vi "Master_ActuatorStates.vi"(8 "error in (no error)":errorcluster) -> (0 "error out":errorcluster, 2 "CurrentActuations":T1={"Pod Power"=FALSE, "Dump Valve"=TRUE, "Brakes"=FALSE, "Clamp"=FALSE, "Pump"=FALSE, "Ignition"=FALSE, "DO6"=FALSE, "DO7"=FALSE, "HighSide"=FALSE, "Precharge"=FALSE, "LowSide"=FALSE, "DO3"=FALSE, "DO4"=FALSE, "DO5"=FALSE, "DO62"=FALSE, "DO72"=FALSE})   [LabVIEW 2018]
doc: "Reads state of actuators and formats it for data stream."
uses:
  Control/TypeDef_DigitalOuts.ctl
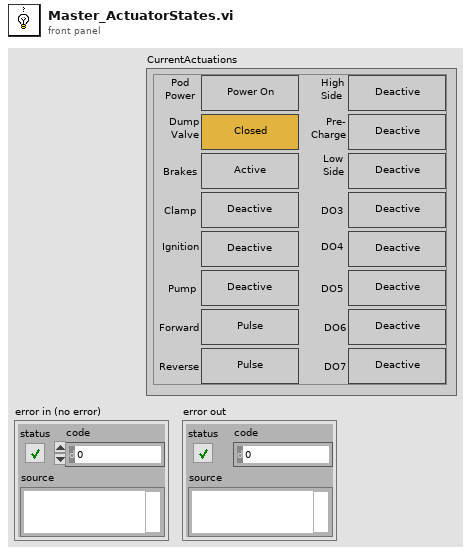
[diagram p1: front panel]
types:
  T1 = typedef "TypeDef_DigitalOuts.ctl" = cluster{"Pod Power":bool, "Dump Valve":bool, "Brakes":bool, "Clamp":bool, "Pump":bool, "Ignition":bool, "DO6":bool, "DO7":bool, "HighSide":bool, "Precharge":bool, "LowSide":bool, "DO3":bool, "DO4":bool, "DO5":bool, "DO62":bool, "DO72":bool}
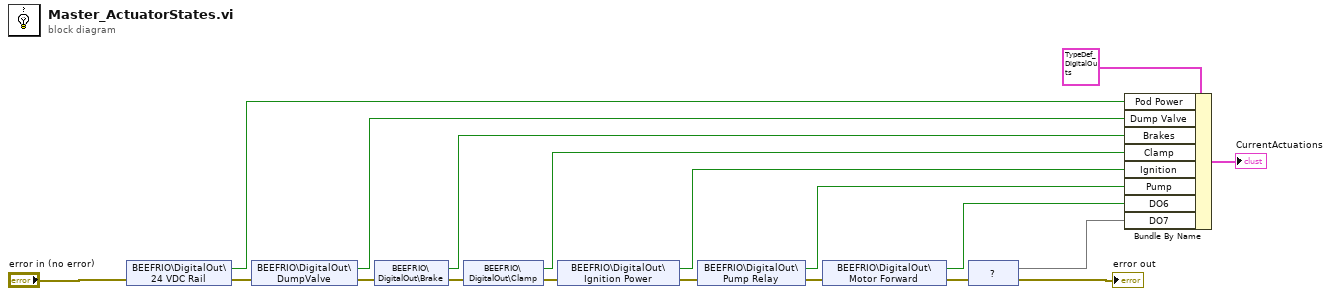
[diagram p0: block diagram]
diagram:
  n1 = shared-variable "BEEFRIO\\DigitalOut\\24 VDC Rail"(error in="error in (no error)") -> (w8:bool, error out=w19:errorcluster)
  n2 = shared-variable "BEEFRIO\\DigitalOut\\DumpValve"(error in=w19) -> (w7:bool, error out=w18:errorcluster)
  n3 = shared-variable "BEEFRIO\\DigitalOut\\Brake"(error in=w18) -> (w6:bool, error out=w17:errorcluster)
  n4 = shared-variable "BEEFRIO\\DigitalOut\\Clamp"(error in=w17) -> (w5:bool, error out=w13:errorcluster)
  n5 = shared-variable "BEEFRIO\\DigitalOut\\Ignition Power"(error in=w13) -> (w4:bool, error out=w16:errorcluster)
  n6 = shared-variable "BEEFRIO\\DigitalOut\\Pump Relay"(error in=w16) -> (w3:bool, error out=w15:errorcluster)
  n7 = shared-variable "BEEFRIO\\DigitalOut\\Motor Forward"(error in=w15) -> (w2:bool, error out=w14:errorcluster)
  n8 = shared-variable "?"(error in=w14) -> (w1, error out=→"error out":errorcluster)
  n9 = Bundle By Name(cluster=T1 {"Pod Power"=FALSE, "Dump Valve"=TRUE, "Brakes"=FALSE, "Clamp"=FALSE, "Pump"=FALSE, "Ignition"=FALSE, "DO6"=FALSE, "DO7"=FALSE, "HighSide"=FALSE, "Precharge"=FALSE, "LowSide"=FALSE, "DO3"=FALSE, "DO4"=FALSE, "DO5"=FALSE, "DO62"=FALSE, "DO72"=FALSE} ("Actuators"), "Pod Power"=w8, "Dump Valve"=w7, "Brakes"=w6, "Clamp"=w5, "Ignition"=w4, "Pump"=w3, "DO6"=w2, "DO7"=w1) -> (→"CurrentActuations":T1)
